vi "更新点位信息表的放料点相对拍照点高度差.vi"(2 "当前产品信息":T2, 3 "锁螺丝点位信息表":string[][](array[string])) -> (0 "更新放料点与拍照点高度差后的锁附点位信息表":string[][](array[string]))   [LabVIEW 2014]
uses:
  ModelInfo.ctl
panel:
  out "每一颗螺丝型号":T1[](array[typedef])
  out "螺杆长度数组":dbl[](array[numeric])
  out "螺帽直径数组":dbl[](array[numeric])
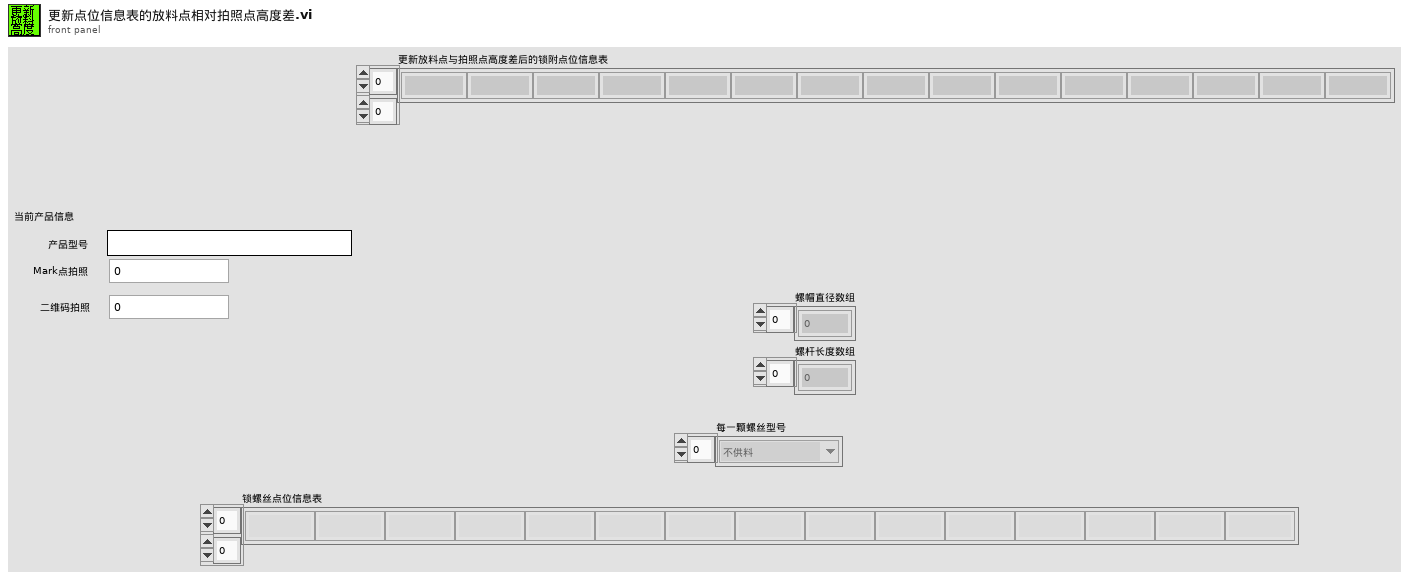
[diagram p1: front panel]
types:
  T1 = typedef "控件-螺丝型号.ctl" = enum16{"不供料", "一字螺丝M2.5*4", "一字螺丝M2.5*6", "一字螺丝M2.5*8", "一字螺丝M2.5*10", "一字螺丝M2.5*12", "一字螺丝M2.5*14", "一字螺丝M2.5*16", "一字螺丝M2.5*18", "一字螺丝M2.5*20", "一字螺丝M3*4", "一字螺丝M3*6", "一字螺丝M3*8", "一字螺丝M3*10", "一字螺丝M3*12", "一字螺丝M3*14", "一字螺丝M3*16", "一字螺丝M3*18", "一字螺丝M3*20", "一字螺丝M4*6", "一字螺丝M4*8", "一字螺丝M4*10", "一字螺丝M4*12", "一字螺丝M4*14", "一字螺丝M4*16", "一字螺丝M4*18", "一字螺丝M4*20", "十字螺丝M2.5*4", "十字螺丝M2.5*6", "十字螺丝M2.5*8", "十字螺丝M2.5*10", "十字螺丝M2.5*12", "十字螺丝M2.5*14", "十字螺丝M2.5*16", "十字螺丝M2.5*18", "十字螺丝M2.5*20", "十字螺丝M3*4", "十字螺丝M3*6", "十字螺丝M3*8", "十字螺丝M3*10", "十字螺丝M3*12", "十字螺丝M3*14", "十字螺丝M3*16", "十字螺丝M3*18", "十字螺丝M3*20", "十字螺丝M4*6", "十字螺丝M4*8", "十字螺丝M4*10", "十字螺丝M4*12", "十字螺丝M4*14", "十字螺丝M4*16", "十字螺丝M4*18", "十字螺丝M4*20"}
  T2 = typedef "ModelInfo.ctl" = cluster{"产品型号":string, "二维码拍照":u32, "Mark点拍照":u32}
  T3 = typedef "锁附点位信息.ctl" = cluster{"点位名称":string, "点位坐标(图纸)":T4, "点位坐标(实际)":T5, "补偿值":T4, "锁附时机械手角度":T6, "放料点相对Mark\n拍照点高度差":dbl, "选择螺丝托盘":enum32{"托盘1", "托盘2", "托盘3", "托盘4", "托盘5", "托盘6", "托盘7", "托盘8"}, "拧紧程式序号":u16, "预锁程式序号":u16, "复锁程式序号":u16, "自动锁螺丝":bool}
  T4 = typedef "XYZPos.ctl" = cluster{"X":dbl, "Y":dbl, "Z":dbl}
  T5 = typedef "XYZRPos.ctl" = cluster{"X":dbl, "Y":dbl, "Z":dbl, "R":dbl}
  T6 = typedef "锁附时机械手角度.ctl" = enum16{"0度", "顺时针90度", "顺时针180度", "逆时针90度", "逆时针180度"}
  T7 = enum32{"托盘1", "托盘2", "托盘3", "托盘4", "托盘5", "托盘6", "托盘7", "托盘8"}
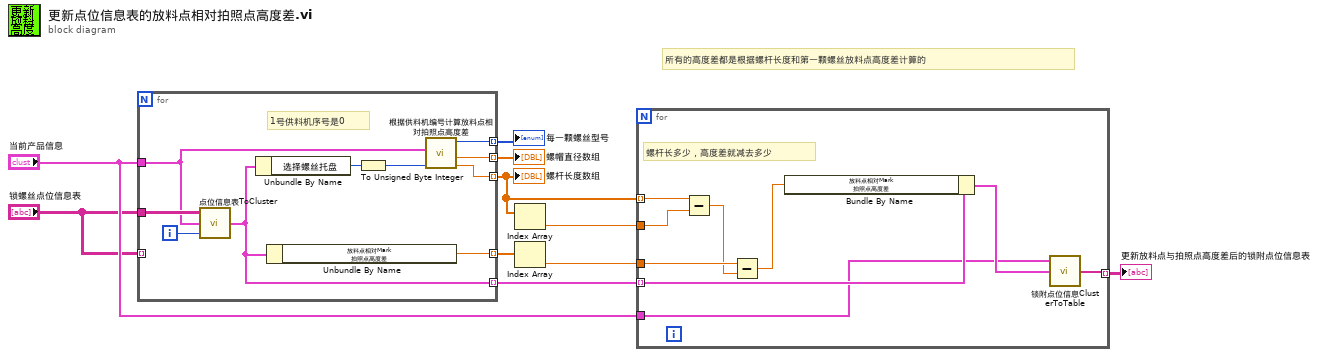
[diagram p0: block diagram]
diagram:
  # "所有的高度差都是根据螺杆长度和第一颗螺丝放料点高度差计算的"
  n1 = for {
    tunnel: "锁螺丝点位信息表" -> [w20]
    tunnel: "当前产品信息" -> [w16]
    tunnel: [w15] -> w10 mode=indexing
    tunnel: [w14] -> w5 mode=indexing
    tunnel: [w13] -> w9 mode=indexing
    tunnel: [w12] -> w8 mode=indexing
    tunnel: [w11] -> w6 mode=indexing
    tunnel: "锁螺丝点位信息表" -> [_] mode=indexing
    i -> [w19]
    # "1号供料机序号是0"
    n2 = call "点位信息表ToCluster.vi"("Row"=w19, "当前产品信息"=w16, "锁附点位信息表"=w20) -> ("锁附点位信息"=w11:T3)
    n3 = Unbundle By Name(w11) -> ("选择螺丝托盘"=w18:T7)
    n4 = Unbundle By Name(w11) -> ("放料点相对Mark\n拍照点高度差"=w12:dbl)
    n5 = To Unsigned Byte Integer(number=w18) -> (unsigned 8bit integer=w17:u8)
    n6 = call "根据供料机编号计算放料点相对拍照点高度差.vi"("供料机编号0~7"=w17, "当前产品信息"=w16) -> ("螺杆长度"=w14:dbl, "螺帽直径"=w15:dbl, "当前供料机螺丝型号"=w13:T1)  [unwired: 7 in]
  }
  "螺帽直径数组" <- w10
  "螺杆长度数组" <- w5
  "每一颗螺丝型号" <- w9
  n7 = Index Array(array=w5) -> (element=w4:dbl)  [unwired: 1 in]
  n8 = Index Array(array=w8) -> (element=w7:dbl)  [unwired: 1 in]
  n9 = for {
    tunnel: [w28] -> w2 mode=indexing
    tunnel: w7 -> [w24]
    tunnel: w6 -> [w27] mode=indexing
    tunnel: w5 -> [w26] mode=indexing
    tunnel: w4 -> [w25]
    tunnel: "当前产品信息" -> [w21]
    # "螺杆长多少，高度差就减去多少"
    n10 = Subtract(x=w26, y=w25) -> (x-y=w23:dbl)
    n11 = Subtract(x=w24, y=w23) -> (x-y=w22:dbl)
    n12 = Bundle By Name(cluster=w27, "放料点相对Mark\n拍照点高度差"=w22) -> (w29:T3)
    n13 = call "锁附点位信息ClusterToTable.vi"("锁附点位信息"=w29, "当前产品信息"=w21) -> ("点位信息表格一行"=w28:string[])  [unwired: 1 in]
  }
  "更新放料点与拍照点高度差后的锁附点位信息表" <- w2
